vi "DB Tools Fetch Recordset Data.vi"   [LabVIEW 2020, in "NI_Database_API.lvlib"]
doc: "Retrieves the data in the recordset identified by the <B>recordset reference</B> input. You can convert each element in the array to its native LabVIEW data type using the Database Variant To Data function. Wire data to the reference input to determine the polymorphic instance to use or manually select the instance."
uses:
  <vilib>/addons/database/NI_Database_API.lvlib
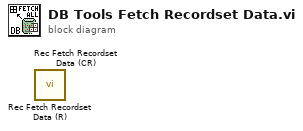
[diagram p0: block diagram]
diagram:
  n1 = call <vilib>:"Rec Fetch Recordset Data (R).vi"() -> ()  [unwired: 5 in, 3 out]
  n2 = call <vilib>:"Rec Fetch Recordset Data (CR).vi"() -> ()  [unwired: 5 in, 3 out]
